vi "AlliGator Update Parameter Map Palette.vi"(8 "error in (no error)":errorcluster, 10 "Parameter Map Display Palette Information":T2 {"Palette Type" items=["Grayscale", "Binary", "Gradient", "Rainbow", "Temperature", "User Defined", "Binary 16 Bit", "Gradient 16 Bit", "Rainbow 16 Bit", "Temperature 16 Bit", "User Defined 16 Bit"]}, 11 "Parameter Map Ctrl Refums":T1) -> (0 "error out":errorcluster)   [LabVIEW 2021, in "AlliGator Parameter Map.lvlib"]
doc: "Updates the color palette of the <B>Decay Fit Parameter Map</B> image."
uses:
  AlliGator Parameter Map.lvlib
  Palette/Image Palette Information.ctl
  Image/Image Display Palette Type.ctl
  AlliGator Parameter Map Control Refnums.ctl
  Image/Image.lvlib
  Palette/Palette.lvlib
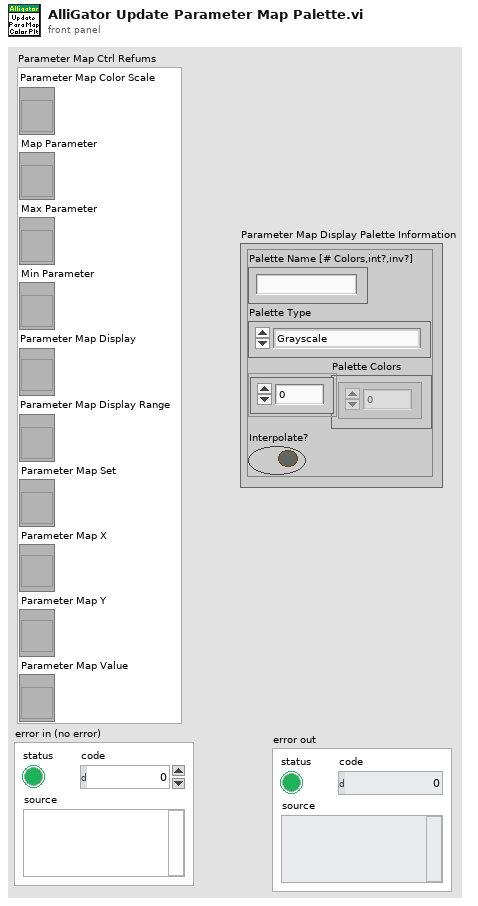
[diagram p1: front panel]
types:
  T1 = typedef "AlliGator Parameter Map.lvlib/AlliGator Parameter Map Control Refnums.ctl" = cluster{"Parameter Map Color Scale":refnum<vi>, "Map Parameter":refnum<vi>, "Max Parameter":refnum<vi>, "Min Parameter":refnum<vi>, "Parameter Map Display":refnum<vi>, "Parameter Map Display Range":refnum<vi>, "Parameter Map Set":refnum<vi>, "Parameter Map X":refnum<vi>, "Parameter Map Y":refnum<vi>, "Parameter Map Value":refnum<vi>}
  T2 = typedef "Palette.lvlib/Image Palette Information.ctl" = cluster{"Palette Name [# Colors,int?,inv?]":string, "Palette Type":T3, "Palette Colors":u32[], "Interpolate?":bool}
  T3 = typedef "Image.lvlib/Image Display Palette Type.ctl" = u32
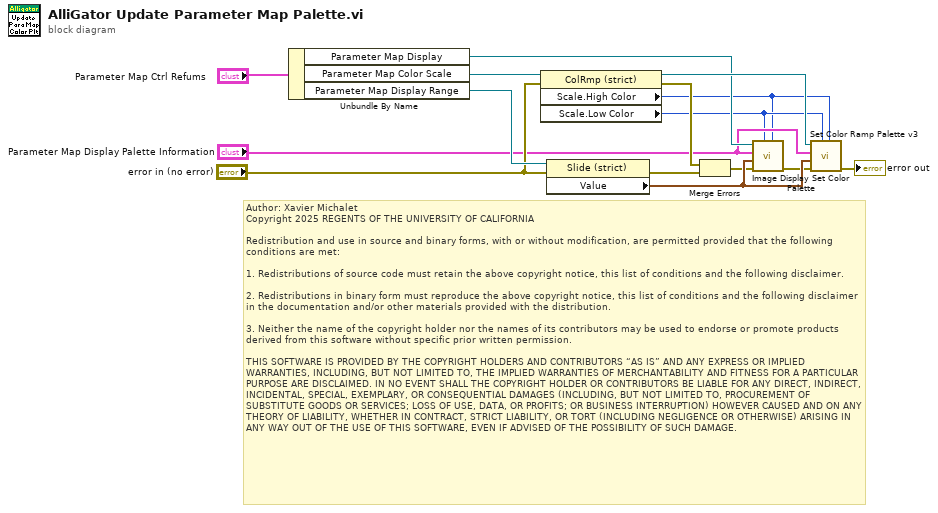
[diagram p0: block diagram]
diagram:
  # "Author: Xavier Michalet\nCopyright 2025 REGENTS OF THE UNIVERSITY OF CALIFORNIA\n\nRedistribution and use in source and binary forms, with or without modification, are permitted provided that the following conditions are met:\n\n1. Redistributions of source code must retain the above copyright notice, this list of conditions and the following disclaimer.\n\n2. Redistributions in binary form must reproduce the above copyright notice, this list of conditions and the following disclaimer in the documentation and/or other materials provided with the distribution.\n\n3. Neither the name of the copyright holder nor the names of its contributors may be used to endorse or promote products derived from this software without specific prior written permission.\n\nTHIS SOFTWARE IS PROVIDED BY THE COPYRIGHT HOLDERS AND CONTRIBUTORS “AS IS” AND ANY EXPRESS OR IMPLIED WARRANTIES, INCLUDING, BUT NOT LIMITED TO, THE IMPLIED WARRANTIES OF MERCHANTABILITY AND FITNESS FOR A PARTICULAR PURPOSE ARE DISCLAIMED. IN NO EVENT SHALL THE COPYRIGHT HOLDER OR CONTRIBUTORS BE LIABLE FOR ANY DIRECT, INDIRECT, INCIDENTAL, SPECIAL, EXEMPLARY, OR CONSEQUENTIAL DAMAGES (INCLUDING, BUT NOT LIMITED TO, PROCUREMENT OF SUBSTITUTE GOODS OR SERVICES; LOSS OF USE, DATA, OR PROFITS; OR BUSINESS INTERRUPTION) HOWEVER CAUSED AND ON ANY THEORY OF LIABILITY, WHETHER IN CONTRACT, STRICT LIABILITY, OR TORT (INCLUDING NEGLIGENCE OR OTHERWISE) ARISING IN ANY WAY OUT OF THE USE OF THIS SOFTWARE, EVEN IF ADVISED OF THE POSSIBILITY OF SUCH DAMAGE."
  n1 = Unbundle By Name("Parameter Map Ctrl Refums") -> ("Parameter Map Display"=w4:refnum<vi>, "Parameter Map Color Scale"=w11:refnum<vi>, "Parameter Map Display Range"=w9:refnum<vi>)
  n2 = property on="Property Node" class="ColRmp (strict)"(reference=w11, error in="error in (no error)") -> (reference out=w10:refnum<vi>, error out=w7:errorcluster, "Scale.High Color"=w1:u32, "Scale.Low Color"=w2:u32)
  n3 = property on="Property Node" class="Slide (strict)"(reference=w9, error in="error in (no error)") -> (error out=w5:errorcluster, "Value"=w14:cluster{dbl, dbl})  [unwired: 1 out]
  n4 = Merge Errors(w7, w5) -> (w6:errorcluster)
  n5 = call "Image Display Set Color Palette.vi"("Image High Color"=w1, "Image Low Color"=w2, "Error In"=w6, "Image Display Range"=w14, "Image Display Palette Information"="Parameter Map Display Palette Information", "Display Image Control Refnum"=w4) -> ("Error Out"=w13:errorcluster)  [unwired: 5 in]
  n6 = call "Set Color Ramp Palette v3.vi"("Image High Color"=w1, "Image Low Color"=w2, "error in (no error)"=w13, "Image Display Range"=w14, "Image Display Palette Information"="Parameter Map Display Palette Information", "ColorRamp in"=w10) -> ("Error Out"=→"error out":errorcluster)  [unwired: 3 in, 2 out]
